vi "basicInfo.vi"(11 "Experiments":T1(array[cluster])) -> (3 "String":string)   [LabVIEW 2020]
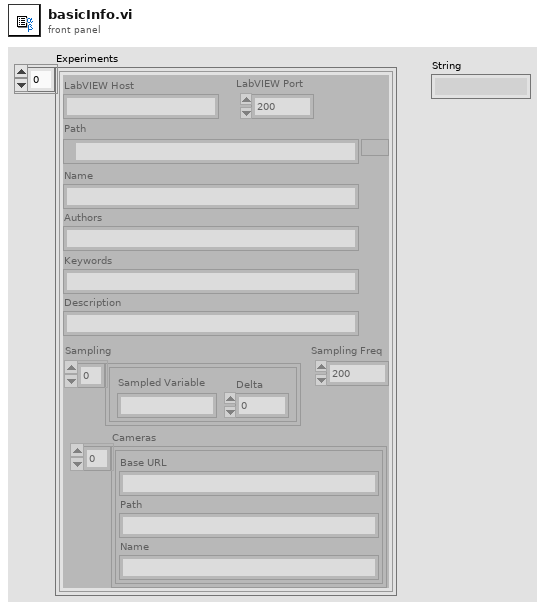
[diagram p1: front panel]
types:
  T1 = cluster{"LabVIEW Host":string, "LabVIEW Port":u32, "Path":path, "Name":string, "Authors":string, "Keywords":string, "Description":string, "Cameras":cluster{"Base URL":string, "Path":string, "Name":string}[], "Sampling":cluster{"Sampled Variable":string, "Delta":dbl}[], "Sampling Freq":u32}[]
  T2 = enum16{"POST_SET", "POST_GET", "SSE_GET", "GET_INFO"}
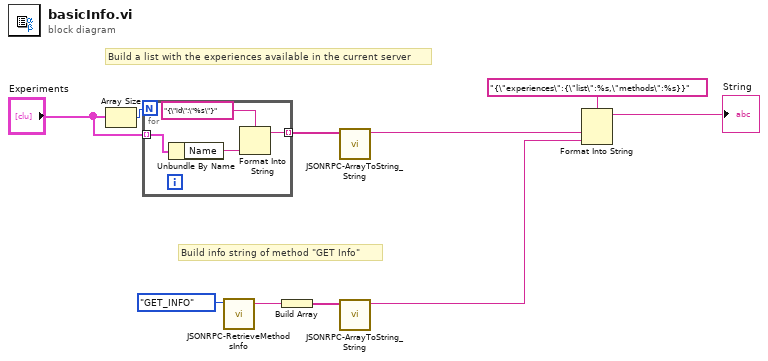
[diagram p0: block diagram]
diagram:
  # "Build a list with the experiences available in the current server"
  # "Build info string of method \"GET Info\""
  n1 = Array Size(array="Experiments") -> (size(s)=w1:i32)
  n2 = for {
    N: w1 -> [_]
    tunnel: "Experiments" -> [w14] mode=indexing
    tunnel: [w11] -> w6 mode=indexing
    n3 = Unbundle By Name(w14) -> ("Name"=w13:string)
    n4 = Format Into String(format string="{\"id\":\"%s\"}", w13) -> (resulting string=w11:string)  [unwired: 2 in, 1 out]
  }
  n5 = call "JSONRPC-RetrieveMethodsInfo.vi"("Method"=T2."GET_INFO") -> ("Output"=w9:string)  [unwired: 10 in]
  n6 = Build Array(w9) -> (w3:string[])
  n7 = call "JSONRPC-ArrayToString_String.vi"("Array"=w6) -> ("Output"=w7:string)  [unwired: 10 in]
  n8 = call "JSONRPC-ArrayToString_String.vi"("Array"=w3) -> ("Output"=w5:string)  [unwired: 10 in]
  n9 = Format Into String(format string="{\"experiences\":{\"list\":%s,\"methods\":%s}}" ("Description"), w7, w5) -> (resulting string=→"String":string)  [unwired: 2 in, 1 out]
